vi "PPFS_Teleop_System_CalcDriveMode.vi"(4 "Traj 6":bool, 6 "Traj 5":bool, 8 "Traj 4":bool, 9 "Traj 3":bool, 10 "Traj 2":bool, 11 "Traj 1":bool) -> (2 "Dirve Mode Changed":bool, 3 "Drive Mode":i32)   [LabVIEW 2019]
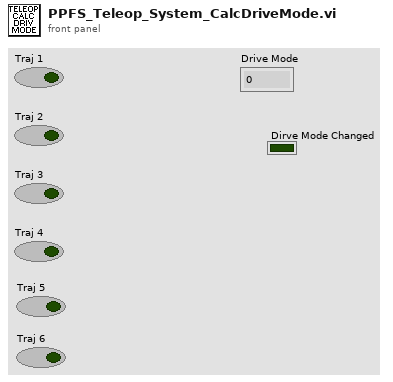
[diagram p1: front panel]
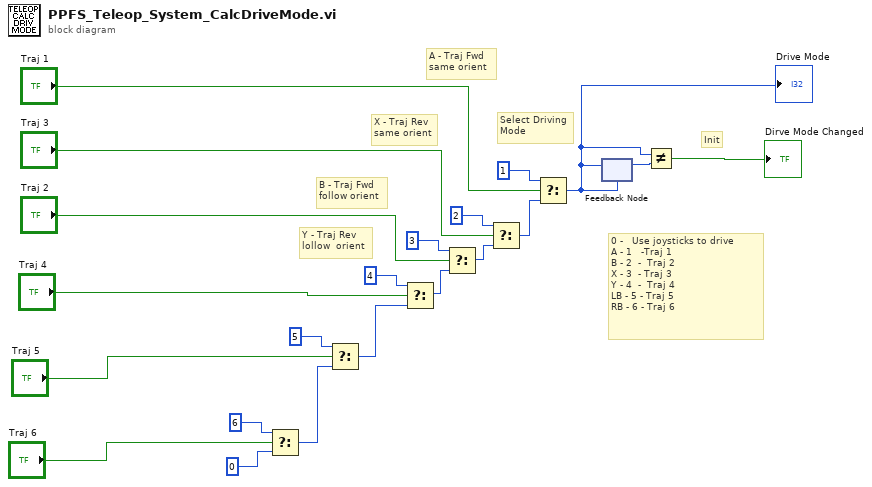
[diagram p0: block diagram]
diagram:
  # "0 -   Use joysticks to drive\nA - 1   -Traj 1\nB - 2  -  Traj 2\nX - 3  - Traj 3\nY - 4  -  Traj 4\nLB - 5 - Traj 5\nRB - 6 - Traj 6"
  # "Init"
  # "Y - Traj Rev \nlollow  orient"
  # "B - Traj Fwd \nfollow orient"
  # "X - Traj Rev\nsame orient"
  # "A - Traj Fwd \nsame orient"
  # "Select Driving\nMode"
  n1 = Select(t=6, s="Traj 6", f=0) -> (s? t:f=w3:i32)
  n2 = Select(t=5, s="Traj 5", f=w3) -> (s? t:f=w4:i32)
  n3 = Select(t=4, s="Traj 4", f=w4) -> (s? t:f=w18:i32)
  n4 = Select(t=3, s="Traj 2", f=w18) -> (s? t:f=w17:i32)
  n5 = Select(t=2, s="Traj 3", f=w17) -> (s? t:f=w14:i32)
  n6 = Select(t=1, s="Traj 1", f=w14) -> (s? t:f=w11:i32)
  "Drive Mode" <- w11
  n7 = feedback #1(w11) -> (w10:i32)
  n8 = feedback-in #1(w11) -> ()
  n9 = Not Equal?(x=w11, y=w10) -> (x != y?=→"Dirve Mode Changed":bool)
